vi "PH_Sequencer.PC PPStatePU.vi"(0 "i ref in":refnum<vi>, 2 "Service Name":string, 3 "State":T1 items=["no info", "off/false/out", "on/true/in", "Failure", "Alarm", "Status 1", "Status 2", "Status 3"], 4 "not linked?":bool, 5 "error in (no error)":errorcluster) -> (14 "i ref out":refnum<vi>, 19 "error out":errorcluster)   [LabVIEW 2014, in "PH_Sequencer.lvlib"]
doc: "This VI writes the state of the PU to own attributes and does some action at first lingange."
uses:
  PH_Sequencer.lvlib
  PH_Basics/PH_StatusHandler/PH_StatusHandler.Status.ctl
  PH_Basics/PH_PowerUnit_BaseClass/PH_PowerUnit_BaseClass.lvlib
  PH_Basics/PH_StatusHandler/PH_StatusHandler.lvlib
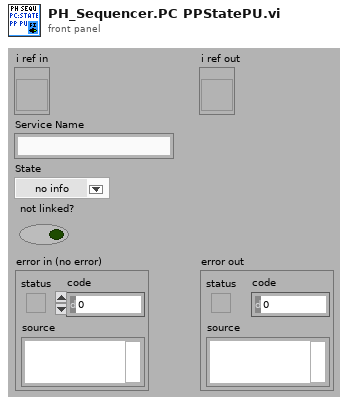
[diagram p1: front panel]
types:
  T1 = typedef "PH_StatusHandler.lvlib/PH_StatusHandler.Status.ctl" = i16
  T2 = typedef "PH_Sequencer.lvlib/PH_Sequencer.Head.ctl" = cluster{"PowerUnit":T3, "GUI Ref":refnum<vi>, "Information":T4, "linked?":bool, "GUI Ref Current Voltage":refnum<vi>}
  T3 = typedef "PH_PP_Common.lvlib/PH_PP_Common.PUs.ctl" = enum16{"no Info", "PA-19mm-1", "PA-19mm-2", "PA-45mm-PILC", "PA-45mm-MAIN", "MA-PU-1", "MA-PU-2", "MA-PU-3", "MA-PU-4", "MA-PU-5", "MA-PU-6", "MA-FR", "MA-PILC", "PA-45mm-DP"}
  T4 = typedef "PH_Sequencer.lvlib/PH_Sequencer.PU Information.ctl" = cluster{"State":T1, "Waiting Time [s]":dbl, "PU State SM":T5, "PU Timeout SM":T5}
  T5 = typedef "PH_PowerUnit_BaseClass.lvlib/PH_PowerUnit_BaseClass.SM States.ctl" = enum16{".", "Stand by", "Switch PU on", "Configure", "Set Default Voltage", "Set STANDBY", "Set READY", "Wait for Shot Cmd", "Open Dump Rods", "Open Ross Relais", "Close Ross Relais", "Switch PSU on", "Switch PSU off", "Charge", "Switch GD Channel on", "Close Dump Rods", "Rods-TO", "RR-TO", "PSU-TO", "Trigger-TO"}
  T6 = typedef "PH_Sequencer.lvlib/PH_Sequencer.i attribute.ctl" = cluster{"GUI Refs":cluster{"Main Off":refnum<vi>, "Fire":refnum<vi>, "Status":refnum<vi>, "Ready":refnum<vi>, "Waiting Time":refnum<vi>, "Timeout":refnum<vi>, "PPMA Ready":refnum<vi>, "Sequencer SM State":refnum<vi>, "PPPA Ready":refnum<vi>, "Calorimeter":refnum<vi>, "Beamline Ready":refnum<vi>, "Clear Beamline":refnum<vi>, "Linkage PPMA Rods":refnum<vi>, "Linkage Current PA":refnum<vi>, "Linkage Current MA":refnum<vi>, "Timing Ready":refnum<vi>, "State Timing":refnum<vi>, "Force Timing":refnum<vi>, "PSDB Shot Comment":refnum<vi>, "State PA Backreflection":refnum<vi>, "Beamline Z6 Ready":refnum<vi>, "Clear Z6 Beamline":refnum<vi>, "Sequence length":refnum<vi>, "Timing Mode":refnum<vi>, "Slow Trigger Settings":refnum<vi>, "Experiment Description":refnum<vi>, "State PSDB":refnum<vi>, "PSDB Ready":refnum<vi>, "Set PSDB Settings":refnum<vi>, "Get PSDB Info":refnum<vi>, "Take Snapshot":refnum<vi>, "Shottype":refnum<vi>, "Experiment":refnum<vi>, "Phase Frontends":refnum<vi>, "PP 45mm PILC in use":refnum<vi>}, "Status Info":cluster{"Machine Status":T1, "WaitingTime":i32, "Timeout":bool}, "Readyness":cluster{"Ready to shot":bool, "PPMA Ready":bool, "PPPA Ready":bool, "BL Ready":bool, "Timing Ready":bool, "BL Z6 Ready":bool, "PSDBReady":bool}, "Instancenames":cluster{"PPMA Rods":string, "PP Current Meas":string, "PH Beamline Chief":string, "PA Backrefl Meas":string, "Z6 Beamline Chief":string}, "Data to read":bool, "Calorimeter":cluster{"Instancename":string, "On":bool, "linked":bool}, "Linkage":cluster{"PPMA Rods":bool, "PP Current Meas":bool, "PHELIX Beamline Chief":bool, "PA Backrefl Meas":bool, "Z6 Beamline Chief":bool}, "Timing":cluster{"Instance":string, "linked":bool, "Status":T1, "Timing Mode":T7, "Slow Trigger Settings":T8, "Info available":cluster{"ext SlowTrigger":bool, "T2":bool, "Mode":bool, "Delay Slow Trigger":bool, "Phase FEs":bool}, "FE Phase":T9}, "Service ID R2S":i32, "PSDB":cluster{"Controller Instance":string, "Controller Status":T1, "Controller linked":bool, "Settings acknowledged":bool, "Current Experiment ID":i16, "Current Shot Type":i16, "Current Comment":string, "Remember Settings":bool, "Write 2 early":bool}, "PSDB Data":cluster{"Main Off?":bool, "Sequence Length":dbl, "Sequence startet":timestamp}, "6P 4Q Positions":cluster{"Instancename":string, "linked":bool, "Position":T10}[], "PUs":T2[]}
  T7 = typedef "PH_Timing.lvlib/PH_Timing.Timing Mode.ctl" = cluster{"T2":i16, "Modeselector":enum32{"10 Hz", "0.5 Hz", "Shot"}}
  T8 = typedef "PH_Timing.lvlib/PH_Timing.Slow Trigger Settings.ctl" = cluster{"Delay":dbl, "externally triggered?":bool}
  T9 = typedef "PH_Timing.lvlib/PH_Timing.Phase FEs.ctl" = cluster{"Phase":dbl}
  T10 = typedef "PH_4_Pos_Selector.lvlib/PH_4_Pos_Selector.Position Selector.ctl" = u16
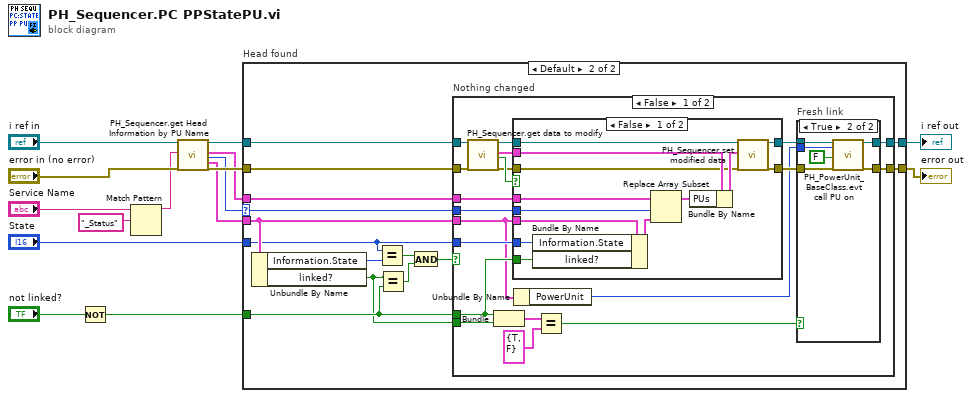
[diagram p0: block diagram]
diagram:
  n1 = Not(x="not linked?") -> (.not. x?=w1:bool)
  n2 = Match Pattern(string="Service Name", regular expression="_Status") -> (before substring=w6:string)  [unwired: 1 in, 3 out]
  n3 = call "PH_Sequencer.get Head Information by PU Name.vi"("i ref in"="i ref in", "PU Instance Name"=w6, "error in (no error)"="error in (no error)") -> ("i ref out"=w9:refnum<vi>, "Heads Information as Array"=w3:T2[], "index of power unit"=w5:i32, "Head Information"=w4:T2, "error out"=w11:errorcluster)  [unwired: 12 in]
  n4 = case "Head found" shown="Default" w5 {
    selector: w5 -> [_ w28]
    tunnel: "State" -> [_ w24]
    tunnel: [w16 w31] -> w14
    tunnel: [w17 w30] -> w13
    tunnel: w11 -> [w16 w26]
    tunnel: w9 -> [w17 w27]
    tunnel: w4 -> [_ w25]
    tunnel: w3 -> [_ w29]
    tunnel: w1 -> [_ w19]
    frame -1 {
    }
    frame Default {
      n5 = Unbundle By Name(w25) -> ("Information.State"=w23:T1, "linked?"=w18:bool)
      n6 = Equal?(x=w24, y=w23) -> (x = y?=w22:bool)
      n7 = Equal?(x=w18, y=w19) -> (x = y?=w21:bool)
      n8 = And(x=w22, y=w21) -> (x .and. y?=w20:bool)
      n9 = case "Nothing changed" shown="False" w20 {
        tunnel: [w34 w75] -> w31
        tunnel: [w36 w76] -> w30
        tunnel: w29 -> [w47 _]
        tunnel: w28 -> [w46 _]
        tunnel: w27 -> [w45 w76]
        tunnel: w26 -> [w44 w75]
        tunnel: w25 -> [w33 _]
        tunnel: w24 -> [w43 _]
        tunnel: w19 -> [w42 _]
        tunnel: w18 -> [w41 _]
        frame False {
          n10 = call "PH_Sequencer.get data to modify.vi"("i ref in"=w45, "error in (no error)"=w44) -> ("i ref out"=w48:refnum<vi>, "i attribute"=w50:T6, "timed out"=w51:bool, "error out"=w49:errorcluster)  [unwired: 14 in]
          n11 = Bundle(w42, "linked?"=w41) -> (w40:cluster{bool, "linked?":bool})  [unwired: 1 in]
          n12 = case shown="False" w51 {
            tunnel: w48 -> [w72 w74]
            tunnel: [w71 w74] -> w37
            tunnel: w49 -> [w61 w73]
            tunnel: [w70 w73] -> w35
            tunnel: w50 -> [w67 _]
            tunnel: w43 -> [w68 _]
            tunnel: w46 -> [w66 _]
            tunnel: w33 -> [w63 _]
            tunnel: w47 -> [w64 _]
            tunnel: w42 -> [w60 _]
            frame False {
              n13 = Bundle By Name(cluster=w63, "Information.State"=w68, "linked?"=w60) -> (w65:T2)
              n14 = Replace Array Subset(array=w64, new element=w65, index=w66) -> (w62:T2[])
              n15 = Bundle By Name(cluster=w67, "PUs"=w62) -> (w69:T6)
              n16 = call "PH_Sequencer.set modified data.vi"("i ref in"=w72, "i attribute"=w69, "error in (no error)"=w61) -> ("i ref out"=w71:refnum<vi>, "error out"=w70:errorcluster)  [unwired: 15 in]
            }
            frame True {
            }
          }
          n17 = Unbundle By Name(w33) -> ("PowerUnit"=w32:T3)
          n18 = Equal?(x=w40, y=cluster{bool, "PU linked":bool} {TRUE, "PU linked"=FALSE}) -> (x = y?=w38:bool)
          n19 = case "Fresh link" shown="True" w38 {
            tunnel: w35 -> [w52 w59]
            tunnel: w37 -> [w53 w58]
            tunnel: [w53 w56] -> w36
            tunnel: [w52 w55] -> w34
            tunnel: w32 -> [_ w54]
            frame False {
            }
            frame True {
              n20 = call "PH_PowerUnit_BaseClass.evt call PU on.vi"("i ref in"=w58, "PowerUnit"=w54, "PU on"=FALSE, "error in (no error)"=w59) -> ("i ref out"=w56:refnum<vi>, "error out"=w55:errorcluster)  [unwired: 14 in]
            }
          }
        }
        frame True {
        }
      }
    }
  }
  "error out" <- w14
  "i ref out" <- w13
